vi "WILT Find Button Press .vi"(8 "error in (no error)":errorcluster, 11 "NewVal":T1[](array[typedef]) {"Night Cycle Count" format="%04d"; "Day Cycle Count" format="%04d"}) -> (0 "error out":errorcluster, 2 "Button Press Happened":bool, 3 "Button Location":i32)   [LabVIEW 2016]
uses:
  Type Definitions/WILT Dryer.ctl
  Type Definitions/WILT Dryer Details.ctl
  Type Definitions/WILT Agilent Channel Definition.ctl
  Type Definitions/WILT DAQ Data.ctl
panel:
  # "Day"
  # "Night"
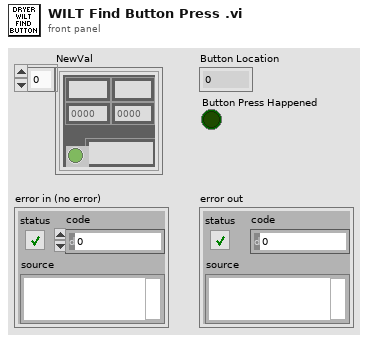
[diagram p1: front panel]
types:
  T1 = typedef "WILT Dryer.ctl" = cluster{"Lab ID":string, "Day Cycle Count":i32, "Station Label":string, "Dryer Details":T2, "Status Color":u32, "Invisible Button":bool, "Night Cycle Count":i32, "Station Index":i32, "Cycle Index":string, "Audit Alert":bool, "Agilent Channel Definition":T3, "DAQ Data":T4}
  T2 = typedef "WILT Dryer Details.ctl" = cluster{"Station":string, "Lab ID":string, "TR Number":string}
  T3 = typedef "WILT Agilent Channel Definition.ctl" = cluster{"Channel":string, "Station":string, "Label":string, "Agilent Station":string, "Data":dbl}
  T4 = typedef "WILT DAQ Data.ctl" = cluster{"L1 Current":dbl, "L2 Current":dbl, "Temperature  Deg F (TC)":dbl, "Volts":dbl, "Volts (208)":dbl, "SW (208)":dbl}
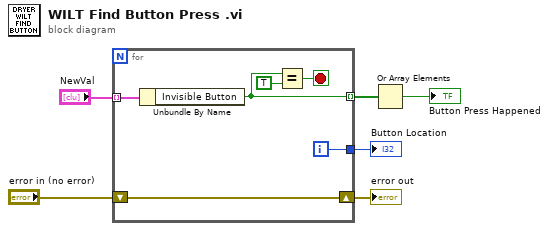
[diagram p0: block diagram]
diagram:
  n1 = for {
    tunnel: "NewVal" -> [w12] mode=indexing
    tunnel: [w9] -> w6
    tunnel: [w8] -> w5 mode=indexing
    shift-right: [w7] -> w4
    shift-left: "error in (no error)" -> [w7]
    i -> [w9]
    stop <- w10 stop-if-true
    n2 = Unbundle By Name(w12) -> ("Invisible Button"=w8:bool)
    n3 = Equal?(x=w8, y=TRUE) -> (x = y?=w10:bool)
  }
  "Button Location" <- w6
  "error out" <- w4
  n4 = Or Array Elements(Boolean array=w5) -> (logical OR=→"Button Press Happened":bool)
